vi "Collection-PED.vi"(8 "error in":errorcluster) -> (0 "error out":errorcluster)   [LabVIEW 2013]
uses:
  <vilib>/Utility/miscctls.llb/LVCursorListTypeDef.ctl
  Collection Support/Controls/PED States.ctl
  Collection Support/Controls/FirstCall.ctl
panel:
  out "Pressure Chart":dynamicdata(graph)
  out "Audio Chart":dynamicdata(graph)
  in  "Exit Button":bool
  in  "Restart Button":bool
  out "Test Type":string
  in  "Settings":bool
  in  "Trial Duration (s)":dbl=10.0 min=0.0 max=15.0 step=1.0 format="%#_13g"
  in  "Max Time":dbl=1.3 min=0.0 max=2.0 format="%#_13g"
  in  "Start Second":dbl=2.5 min=1.0 max=2.5 step=0.1 format="%#_13g"
  in  "Interruptions":i32 min=0 max=10 step=1
  in  "Delay":u32 max=1000 step=50
  in  "Min Time":dbl=0.8 min=0.0 max=1.0 step=0.1 format="%#_13g"
  out "SPL Chart":cluster{"Y":dbl[], "Y":dbl[]}[](graph)
  out "Saving Data":bool
  out "Countdown":dbl format="%#.0g"
  in  "START/STOP":bool
  in  "Stopped?":bool
  out "GO/STOP":bool
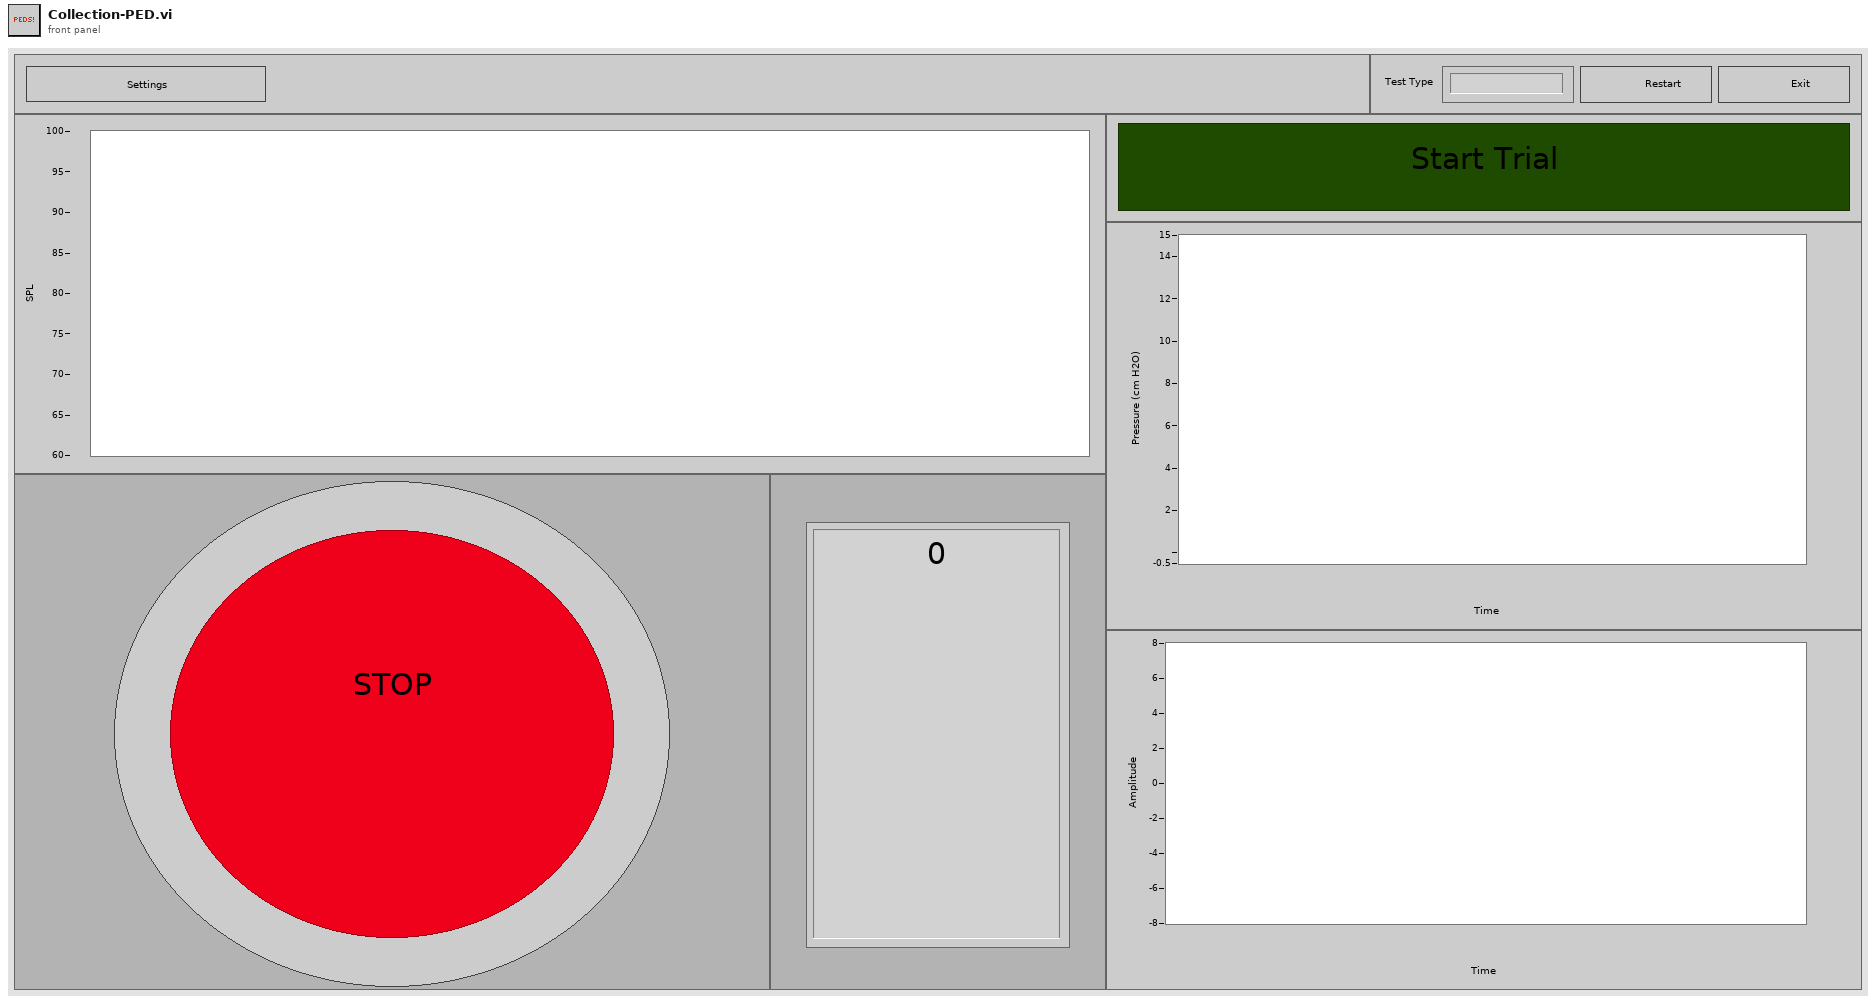
[diagram p1: front panel]
types:
  T1 = enum16{"open", "replace", "create", "open or create", "replace or create", "replace or create with confirmation"}
  T2 = typedef "LVCursorListTypeDef.ctl" = cluster{"Name":string, "Color":u32, "Style":u8, "Point Style":u8, "Name Visible":bool, "Allow Drag":bool, "Cursor Mode":u32, "Plot":i32, "Index":i32, "Position":cluster{"X":dbl, "Y":dbl}, "X Scale":u32, "Y Scale":u32, "Watch Plots":i32[], "Watch All Plots":bool, "Plot Area":i32, "Label Offset":cluster{"X":dbl, "Y":dbl}}[]
  T3 = typedef "PED States.ctl" = enum16{"Initialize", "Wait", "Record", "Save", "Reset", "Exit"}
  T4 = typedef "FirstCall.ctl" = enum16{"First", "After"}
  T5 = typedef "Mech-Labial Test Types.ctl" = u16
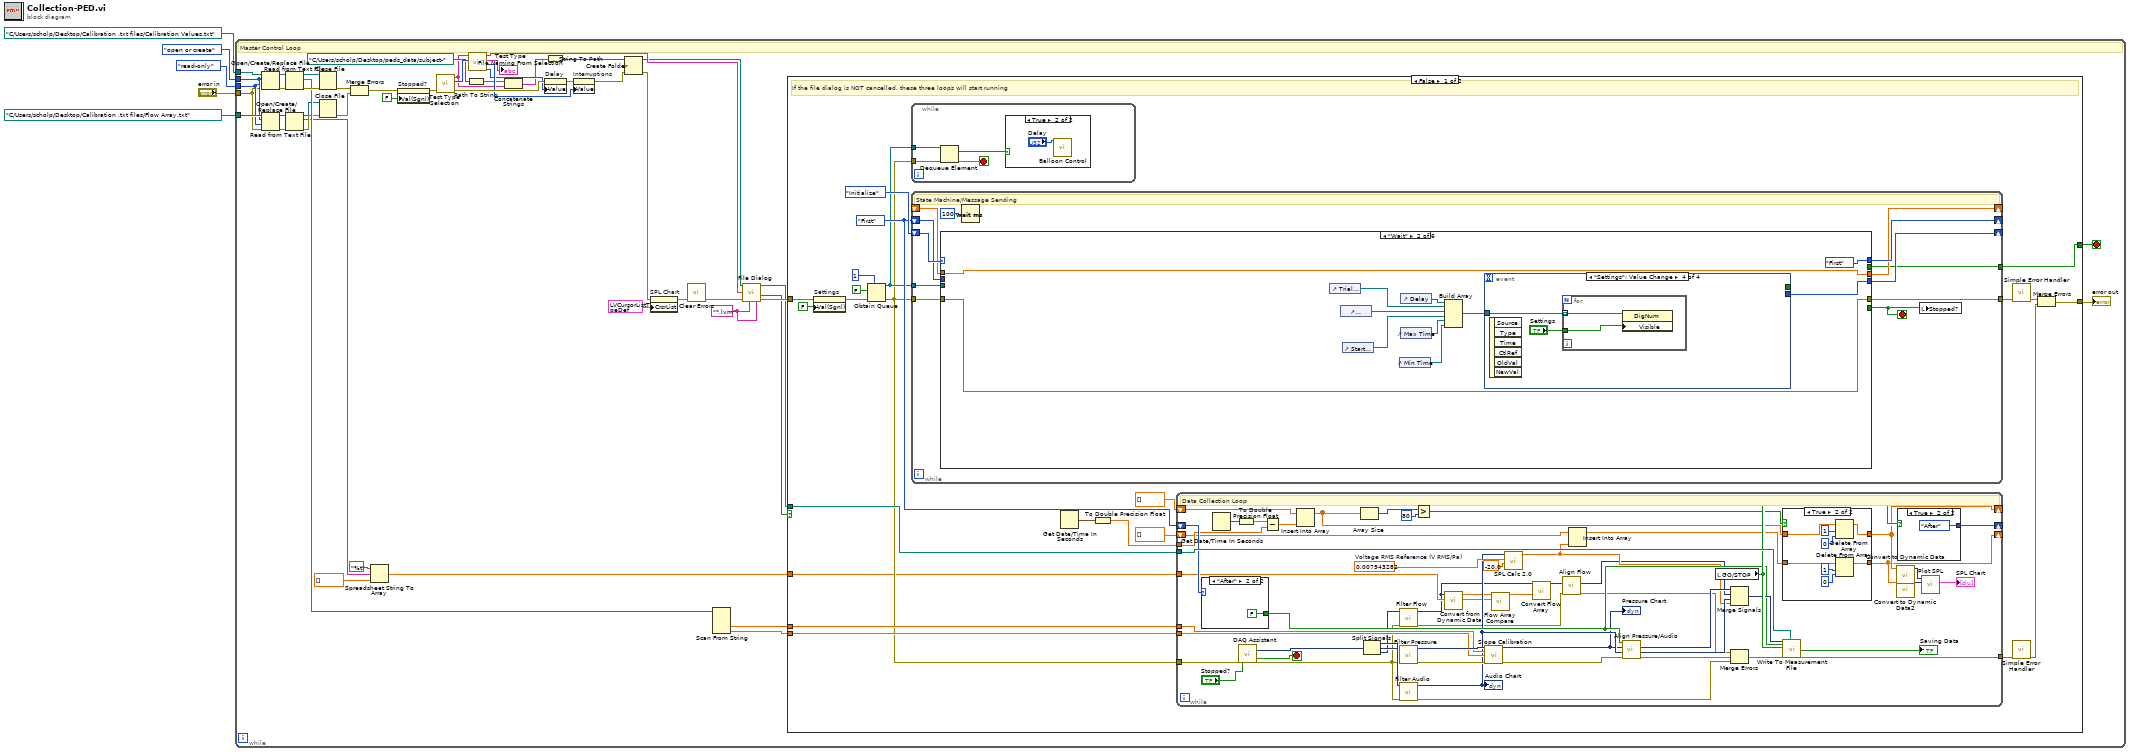
[diagram p0: block diagram]
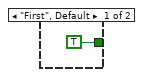
[diagram p4: hidden frame]
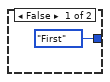
[diagram p5: hidden frame]
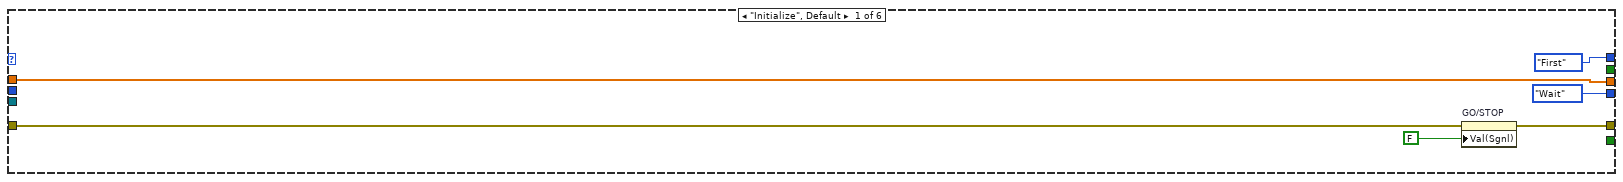
[diagram p6: hidden frame]
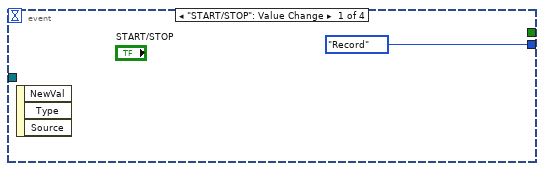
[diagram p7: hidden frame]
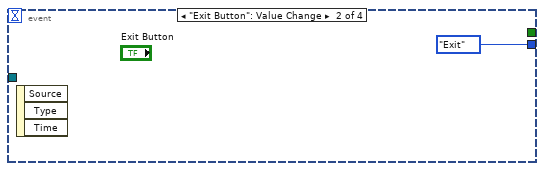
[diagram p8: hidden frame]
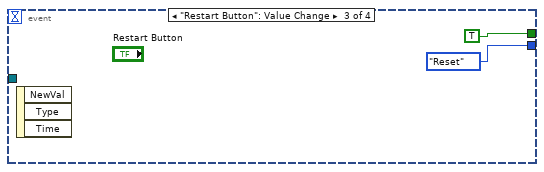
[diagram p9: hidden frame]
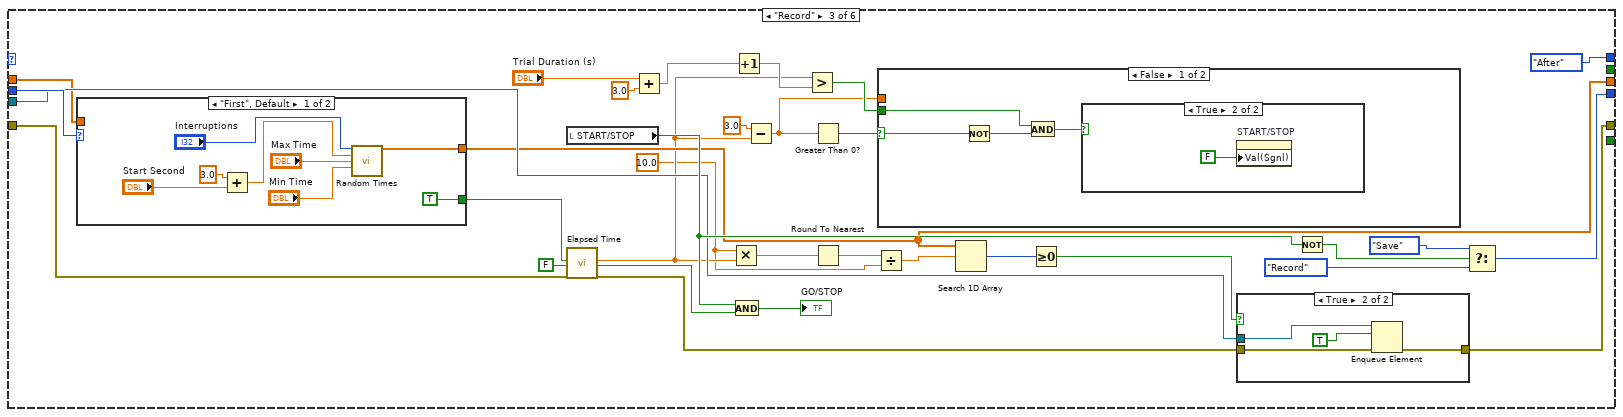
[diagram p10: hidden frame]
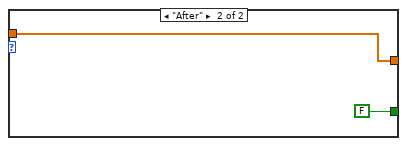
[diagram p12: hidden frame]
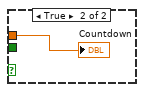
[diagram p14: hidden frame]
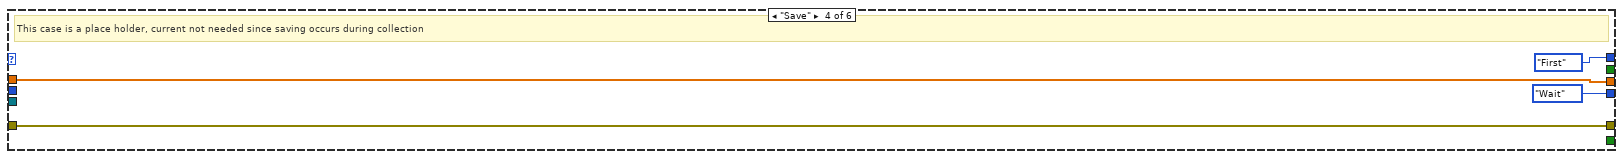
[diagram p15: hidden frame]
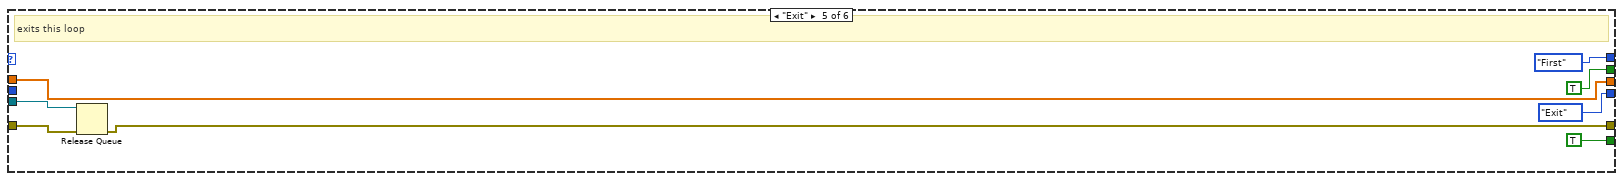
[diagram p16: hidden frame]
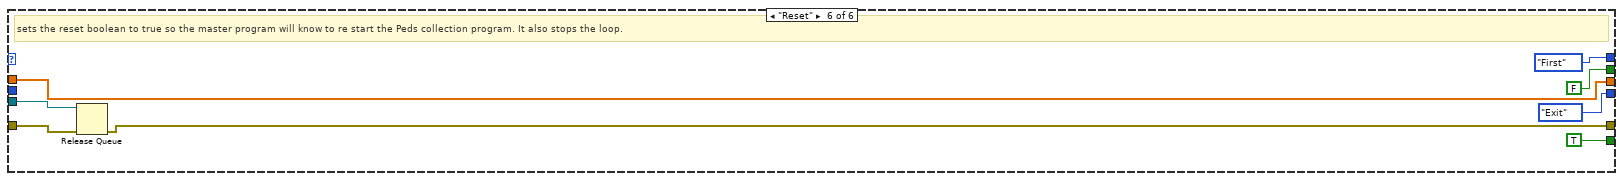
[diagram p17: hidden frame]
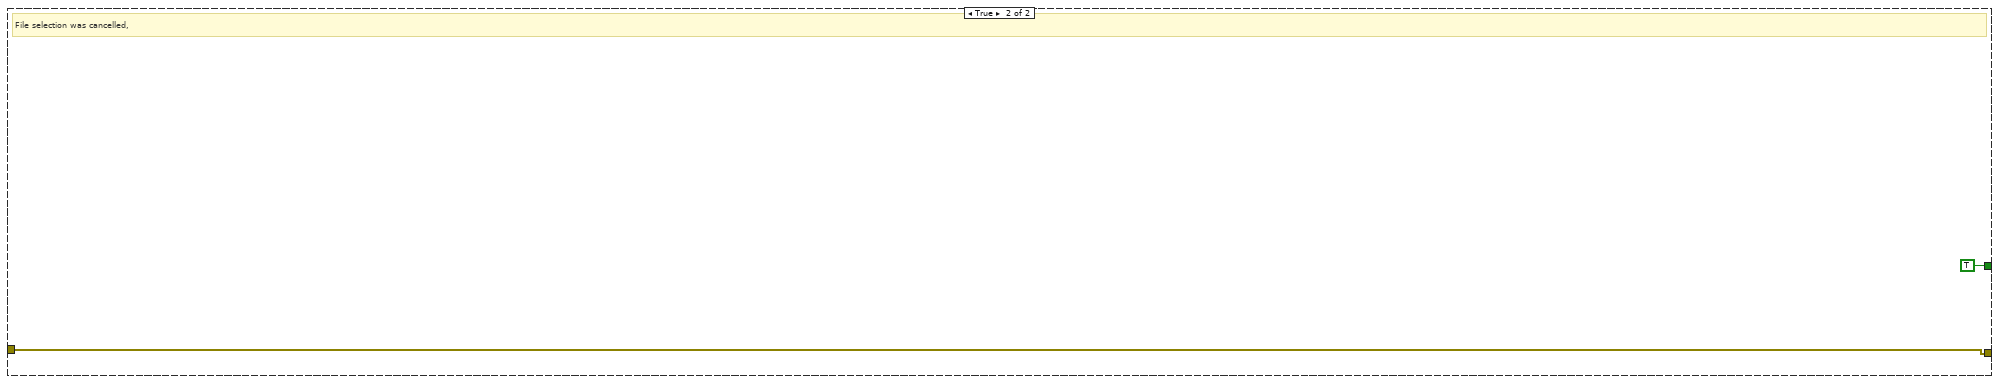
[diagram p18: hidden frame]
diagram:
  n1 = while {
    tunnel: T1."open or create" ("operation (0:open)") -> [w15]
    tunnel: enum16{"read/write", "read-only", "write-only"}."read-only" ("access (0:read/write)") -> [w14]
    tunnel: path "C:/Users/scholp/Desktop/Calibration .txt files/Calibration Values.txt" ("file path (use dialog)") -> [w47]
    tunnel: "error in" -> [w13]
    tunnel: path "C:/Users/scholp/Desktop/Calibration .txt files/Flow Array.txt" ("file path (use dialog)") -> [w16]
    stop <- w37 stop-if-true
    w52 = "*.lvm" ("pattern label")
    # "Master Control Loop"
    n2 = Open/Create/Replace File(file path (use dialog)=w47, error in=w13, operation (0:open)=w15, access (0:read/write)=w14) -> (refnum out=w48:refnum<file>, error out=w50:errorcluster)  [unwired: 2 in, 1 out]
    n3 = Open/Create/Replace File(file path (use dialog)=w16, error in=w13, operation (0:open)=w15, access (0:read/write)=w14) -> (refnum out=w18:refnum<file>, error out=w20:errorcluster)  [unwired: 2 in, 1 out]
    n4 = Read from Text File(file (use dialog)=w48, error in=w50) -> (refnum out=w46:refnum<file>, text=w45:string, error out=w49:errorcluster)  [unwired: 2 in, 1 out]
    n5 = Read from Text File(file (use dialog)=w18, error in=w20) -> (refnum out=w17:refnum<file>, text=w8:string, error out=w19:errorcluster)  [unwired: 2 in, 1 out]
    n6 = Close File(refnum=w46, error in=w49) -> (error out=w11:errorcluster)  [unwired: 1 out]
    n7 = Close File(refnum=w17, error in=w19) -> (error out=w10:errorcluster)  [unwired: 1 out]
    n8 = Merge Errors(w11, w10) -> (w12:errorcluster)
    n9 = Spreadsheet String To Array(format string="%t", spreadsheet string=w8, array type (2D Dbl)=dbl[] []) -> (array=w7:dbl[])  [unwired: 1 in]
    n10 = property on="Stopped?" class="Bool (strict)"(error in=w12, "Val(Sgnl)"=FALSE ("Value (Signaling)")) -> (error out=w40:errorcluster)  [unwired: 1 in, 1 out]
    n11 = call "Test Type Selection.vi"("Error In"=w40) -> ("Error Out"=w39:errorcluster, "Test Type Out"=w32:T5, "Subject Out"=w28:string)  [unwired: 8 in]
    n12 = Path To String(path=path "C:/Users/scholp/Desktop/peds_data/subject-" ("start path")) -> (string=w29:string)
    n13 = call "File Naming From Selection.vi"("Test Type In"=w32, "Subject In"=w28) -> ("Delay"=w33:u32, "Interruptions"=w34:u32, "Test Type"=→"Test Type":string, "File Name"=w36:string)  [unwired: 6 in]
    n14 = Concatenate Strings(w29, w28) -> (w27:string)
    n15 = property on="Delay" class="DigNum (strict)"(error in=w39, "Value"=w33) -> (error out=w38:errorcluster)  [unwired: 1 in, 1 out]
    n16 = String To Path(string=w27) -> (path=w26:path)
    n17 = property on="Interruptions" class="DigNum (strict)"(error in=w38, "Value"=w34) -> (error out=w24:errorcluster)  [unwired: 1 in, 1 out]
    n18 = Create Folder(path (use dialog)=w26, error in=w24) -> (created path=w31:path, error out=w22:errorcluster)  [unwired: 1 in, 1 out]
    n19 = property on="SPL Chart" class="XYGraph (strict)"(error in=w22, "CrsrList"=T2 [{"Name"="Upper", "Color"=16860, "Style"=6, "Point Style"=6, "Name Visible"=TRUE, "Allow Drag"=TRUE, "Cursor Mode"=0, "Plot"=0, "Index"=0, "Position"={"X"=4.012670393065205, "Y"=89.47406993320811}, "X Scale"=0, "Y Scale"=0, "Watch Plots"=[], "Watch All Plots"=FALSE, "Plot Area"=0, "Label Offset"={"X"=-0.0013496383482243246, "Y"=198885117671824.3}}, {"Name"="Lower", "Color"=6618880, "Style"=6, "Point Style"=13, "Name Visible"=TRUE, "Allow Drag"=TRUE, "Cursor Mode"=0, "Plot"=0, "Index"=0, "Position"={"X"=1.9573651669874723, "Y"=85.30922361500785}, "X Scale"=0, "Y Scale"=0, "Watch Plots"=[], "Watch All Plots"=FALSE, "Plot Area"=0, "Label Offset"={"X"=0.0011253990502635425, "Y"=1813042855982289.8}}] ("Cursor List")) -> (error out=w21:errorcluster)  [unwired: 1 in, 1 out]
    n20 = call <vilib>:"Clear Errors.vi"("error in (no error)"=w21) -> ("error out"=w25:errorcluster)  [unwired: 6 in]
    n21 = Scan From String(input string=w45) -> (output 1=w44:dbl, output 2=w43:dbl)  [unwired: 5 in, 3 out]
    n22 = call "File Dialog"("start path"=w31, "default name"=w36, "error in"=w25, "pattern (all files)"=w52, "pattern label"=w52) -> ("selected path"=w53:path, "cancelled"=w42:bool, "error out"=w54:errorcluster)  [unwired: 7 in, 1 out]
    n23 = case shown="False" w42 {
      tunnel: w54 -> [w61 w263]
      tunnel: w53 -> [w73 _]
      tunnel: w44 -> [w70 _]
      tunnel: w43 -> [w69 _]
      tunnel: [w66 w263] -> w41
      tunnel: [w65 TRUE] -> w37
      tunnel: w7 -> [w55 _]
      frame False {
        w74 = FirstCall."First"
        # "If the file dialog is NOT cancelled, these three loops will start running"
        n24 = property on="Settings" class="Bool (strict)"(error in=w61, "Val(Sgnl)"=FALSE ("Value (Signaling)")) -> (error out=w60:errorcluster)  [unwired: 1 in, 1 out]
        n25 = Obtain Queue(max queue size (-1, unlimited)=1, element data type=FALSE, error in (no error)=w60) -> (queue out=w64:refnum<queue>, error out=w63:errorcluster)  [unwired: 2 in, 1 out]
        n26 = while {
          tunnel: w64 -> [w81]
          tunnel: w63 -> [w80]
          stop <- w79 stop-if-true
          n27 = Dequeue Element(queue=w81, error in (no error)=w80) -> (element=w78:bool, error out=w79:errorcluster)  [unwired: 1 in, 2 out]
          n28 = case shown="True" w78 {
            frame False {
            }
            frame True {
              n29 = call "Balloon Control.vi"("Delay (ms)"="Delay") -> ()  [unwired: 11 in]
            }
          }
        }
        n30 = while {
          shift-right: [w163] -> _
          shift-left: PED_States."Initialize" -> [w162]
          tunnel: w64 -> [w159]
          tunnel: w63 -> [w161]
          shift-right: [w158] -> _
          shift-left: w74 -> [w160]
          tunnel: [w156] -> w71
          shift-right: [w153] -> _
          shift-left: _ -> [w154]
          tunnel: [w152] -> w65
          stop <- w157 stop-if-true
          # "State Machine/Message Sending"
          n31 = case shown="\"Wait\"" w162 {
            tunnel: [_ _ _ _ TRUE TRUE] -> w157
            tunnel: [PED_States."Wait" ("f") w180 w205 PED_States."Wait" ("element") PED_States."Exit" ("element") PED_States."Exit" ("element")] -> w163
            tunnel: w161 -> [w164 w177 w211 w243 w251 w256]
            tunnel: w160 -> [_ _ w207 _ _ _]
            tunnel: w159 -> [_ _ w202 _ w250 w255]
            tunnel: [FirstCall."First" FirstCall."First" FirstCall."After" FirstCall."First" FirstCall."First" FirstCall."First"] -> w158
            tunnel: [w167 w178 w199 w242 w247 w261] -> w153
            tunnel: [w165 w177 w201 w243 w248 w257] -> w156
            tunnel: w154 -> [w167 w178 w198 w242 w247 w261]
            tunnel: [_ _ _ _ TRUE FALSE] -> w152
            frame "Initialize", Default {
              n32 = property on="GO/STOP" class="Bool (strict)"(error in=w164, "Val(Sgnl)"=FALSE ("Value (Signaling)")) -> (error out=w165:errorcluster)  [unwired: 1 in, 1 out]
            }
            frame "Wait" {
              n33 = control-ref of="Trial Duration (s)"() -> (w172:refnum<vi>)
              n34 = control-ref of="Interruptions"() -> (w173:refnum<vi>)
              n35 = control-ref of="Start Second"() -> (w174:refnum<vi>)
              n36 = control-ref of="Min Time"() -> (w176:refnum<vi>)
              n37 = control-ref of="Delay"() -> (w171:refnum<vi>)
              n38 = control-ref of="Max Time"() -> (w175:refnum<vi>)
              n39 = Build Array(w171, w172, w173, w174, w175, w176) -> (w170:refnum<vi>[])
              n40 = event shown="[3] \"Settings\": Value Change" {
                selector: _ -> [_ _ _ _]
                dyn-events: _ -> [_ _ _ _]
                timeout: _ -> [_ _ _ _]
                tunnel: [PED_States."Record" ("element") PED_States."Exit" ("element") PED_States."Reset" ("element") _] -> w180
                tunnel: [_ _ TRUE _] -> _
                tunnel: w170 -> [_ _ _ w186]
                event "START/STOP": Value Change {
                  n41 = event-data() -> ()  [unwired: 1 in, 3 out]
                }
                event "Exit Button": Value Change {
                  n42 = event-data() -> ()  [unwired: 1 in, 3 out]
                }
                event "Restart Button": Value Change {
                  n43 = event-data() -> ()  [unwired: 1 in, 3 out]
                }
                event "Settings": Value Change {
                  n44 = event-data() -> ()  [unwired: 1 in, 6 out]
                  n45 = for {
                    tunnel: w186 -> [w188] mode=indexing
                    tunnel: "Settings" -> [w187]
                    n46 = property class="DigNum"(reference=w188, "Visible"=w187) -> ()  [unwired: 1 in, 2 out]
                  }
                }
              }
            }
            frame "Record" {
              w190 = 10.0 ("x")
              n47 = case shown="\"First\", Default" w207 {
                tunnel: [TRUE FALSE] -> w208
                tunnel: [w230 w234] -> w199
                tunnel: w198 -> [_ w234]
                frame "First", Default {
                  n48 = Add(x=3.0, y="Start Second") -> (x+y=w228:dbl)
                  n49 = call "Random Times.vi"("Number of Interruptions"="Interruptions", "Start Second"=w228, "Longest Gap"="Max Time", "Shortest Gap"="Min Time") -> ("Interruption TImes"=w230:dbl[])  [unwired: 10 in, 1 out]
                }
                frame "After" {
                }
              }
              n50 = local read "START/STOP"() -> (w212:bool)
              n51 = call "Elapsed Time"("Reset"=w208, "Auto Reset"=FALSE, "error in (no error)"=w211) -> ("Elapsed Time (s)"=w192:dbl, "Time has Elapsed"=w214:bool, "error out"=w203:errorcluster)  [unwired: 9 in, 5 out]
              n52 = Add(x="Trial Duration (s)", y=3.0) -> (x+y=w195:dbl)
              n53 = Multiply(x=w190, y=w192) -> (x*y=w193:dbl)
              n54 = And(x=w212, y=w214) -> (x .and. y?=→"GO/STOP":bool)
              n55 = Increment(x=w195) -> (x+1=w197:dbl)
              n56 = Subtract(x=3.0, y=w192) -> (x-y=w215:dbl)
              n57 = Greater?(x=w192, y=w197) -> (0:w217:bool)
              n58 = Greater Than 0?(x=w215) -> (x > 0?=w218:bool)
              n59 = Round To Nearest(number=w193) -> (nearest integer value=w191:dbl)
              n60 = Divide(x=w191, y=w190) -> (x/y=w189:dbl)
              n61 = case shown="False" w218 {
                selector: w218 -> [w237 _]
                tunnel: w215 -> [_ w241]
                tunnel: w217 -> [w239 _]
                frame False {
                  n62 = Not(x=w237) -> (.not. x?=w236:bool)
                  n63 = And(x=w239, y=w236) -> (x .and. y?=w238:bool)
                  n64 = case shown="True" w238 {
                    frame False {
                    }
                    frame True {
                      n65 = property on="START/STOP" class="Bool (strict)"("Val(Sgnl)"=FALSE ("Value (Signaling)")) -> ()  [unwired: 2 in, 2 out]
                    }
                  }
                }
                frame True {
                  "Countdown" <- w241
                }
              }
              n66 = Search 1D Array(1D array=w199, element=w189) -> (index of element=w204:i32)  [unwired: 1 in]
              n67 = Greater Or Equal To 0?(x=w204) -> (x >= 0?=w200:bool)
              n68 = case shown="True" w200 {
                tunnel: [w221 w225] -> w201
                tunnel: w203 -> [w221 w224]
                tunnel: w202 -> [_ w223]
                frame False {
                }
                frame True {
                  n69 = Enqueue Element(queue=w223, element=TRUE, error in (no error)=w224) -> (error out=w225:errorcluster)  [unwired: 1 in, 2 out]
                }
              }
              n70 = Not(x=w212) -> (.not. x?=w210:bool)
              n71 = Select(t=PED_States."Save" ("f"), s=w210, f=PED_States."Record") -> (s? t:f=w205:T3)
            }
            frame "Save" {
              # "This case is a place holder, current not needed since saving occurs during collection"
            }
            frame "Exit" {
              # "exits this loop"
              n72 = Release Queue(queue=w250, error in (no error)=w251) -> (error out=w248:errorcluster)  [unwired: 1 in, 2 out]
            }
            frame "Reset" {
              # "sets the reset boolean to true so the master program will know to re start the Peds collection program. It also stops the loop."
              n73 = Release Queue(queue=w255, error in (no error)=w256) -> (error out=w257:errorcluster)  [unwired: 1 in, 2 out]
            }
          }
          n74 = Wait (ms)(milliseconds to wait=u32 100) -> ()  [unwired: 1 out]
          n75 = local write "Stopped?"(w157) -> ()
        }
        n76 = Get Date/Time In Seconds() -> (seconds since 1Jan1904=w59:timestamp)
        n77 = To Double Precision Float(number=w59) -> (double precision float=w58:dbl)
        n78 = while {
          tunnel: w63 -> [w134]
          shift-right: [w132] -> _
          shift-left: w74 -> [w127]
          tunnel: w73 -> [w129]
          tunnel: [w128] -> w72
          tunnel: w70 -> [w131]
          tunnel: w69 -> [w130]
          tunnel: w58 -> [w106]
          shift-right: [w102] -> _
          shift-left: dbl[] [] -> [w105]
          shift-right: [w96] -> _
          shift-left: dbl[] [] -> [w103]
          tunnel: w55 -> [w88]
          stop <- w135 stop-if-true
          w113 = 0.007943282  # Voltage RMS Reference (V RMS/Pa)
          # "Data Collection Loop"
          n79 = case shown="\"After\"" w127 {
            tunnel: [TRUE FALSE] -> w114
            frame "First", Default {
            }
            frame "After" {
            }
          }
          n80 = Get Date/Time In Seconds() -> (seconds since 1Jan1904=w110:timestamp)
          n81 = To Double Precision Float(number=w110) -> (double precision float=w107:dbl)
          n82 = call "DAQ Assistant"("error in"=w134, "stop (F)"="Stopped?") -> ("data"=w124:dynamicdata, "stopped"=w135:bool, "error out"=w92:errorcluster)  [unwired: 14 in, 1 out]
          n83 = Subtract(x=w107, y=w106) -> (x-y=w104:dbl)
          n84 = Insert Into Array(array=w105, new element=w104) -> (w101:dbl[])  [unwired: 1 in]
          n85 = Array Size(array=w101) -> (size(s)=w98:i32)
          n86 = Split Signals(w124) -> (w123:dynamicdata, w122:dynamicdata, w93:dynamicdata)  [unwired: 3 in]
          n87 = call "Filter Flow"("error in (no error)"=w92, "Signal"=w93) -> ("error out"=w84:errorcluster, "Filtered Signal"=w87:dynamicdata)  [unwired: 8 in]
          n88 = call "Filter Pressure"("error in (no error)"=w92, "Signal"=w122) -> ("error out"=w136:errorcluster, "Filtered Signal"=w137:dynamicdata)  [unwired: 8 in]
          n89 = call "Filter Audio"("error in (no error)"=w92, "Signal"=w123) -> ("error out"=w118:errorcluster, "Filtered Signal"=w95:dynamicdata)  [unwired: 8 in]
          "Audio Chart" <- w95
          n90 = Greater?(x=w98, y=80) -> (0:w99:bool)
          n91 = call "Convert from Dynamic Data"("Dynamic Data Type"=w87) -> ("Array"=w89:dbl[])  [unwired: 3 in]
          n92 = call "Slope Calibration.vi"("Voltage"=w137, "Slope"=w131, "Intercept"=w130, "error in (no error)"=w136) -> ("Result"=w94:dynamicdata, "error out"=w120:errorcluster)  [unwired: 10 in]
          "Pressure Chart" <- w94
          n93 = call "Flow Array Compare.vi"("Flow Array in"=w88, "Array in"=w89) -> ("Array out"=w90:dbl[])  [unwired: 9 in]
          n94 = call "SPL Calc 2.0.vi"("Gain"=-20.0, "Voltage RMS Reference (V RMS/Pa)"=w113, "Dynamic Data"=w95) -> ("SPL"=w91:dbl)  [unwired: 8 in]
          n95 = call "Convert Flow Array.vi"("Voltage"=w87, "Array - Numeric"=w90) -> ("Result"=w86:dynamicdata)  [unwired: 12 in, 1 out]
          n96 = call "Align Flow"("error in (no error)"=w84, "Signals"=w86) -> ("error out"=w83:errorcluster, "Resampled Signals"=w85:dynamicdata)  [unwired: 7 in, 1 out]
          n97 = Insert Into Array(array=w103, new element=w91) -> (w97:dbl[])  [unwired: 1 in]
          n98 = call "Align Pressure/Audio"("error in (no error)"=w120, "Signals 2"=w95, "Signals"=w94, "Reset"=w114) -> ("error out"=w119:errorcluster, "Resampled Signals 2"=w117:dynamicdata, "Resampled Signals"=w121:dynamicdata)  [unwired: 5 in]
          n99 = local read "GO/STOP"() -> (w125:bool)
          n100 = Merge Signals(w121, w85, w117, w91) -> (w116:dynamicdata)
          n101 = Merge Errors(w83, w119, w118) -> (w115:errorcluster)
          n102 = case shown="True" w99 {
            tunnel: w101 -> [w139 w147]
            tunnel: [w139 w146] -> w102
            tunnel: w97 -> [w138 w141]
            tunnel: [w138 w140] -> w96
            frame False {
            }
            frame True {
              n103 = Delete From Array(array=w147, length=1, index=0) -> (array with subset deleted=w146:dbl[])  [unwired: 1 out]
              n104 = Delete From Array(array=w141, length=1, index=0) -> (array with subset deleted=w140:dbl[])  [unwired: 1 out]
            }
          }
          n105 = call "Write To Measurement File"("Signals"=w116, "Reset"=w114, "Enable"=w125, "error in (no error)"=w115, "Filename"=w129) -> ("Saving Data"=→"Saving Data":bool, "error out"=w128:errorcluster)  [unwired: 12 in, 1 out]
          n106 = call "Convert to Dynamic Data"("Array"=w102) -> ("Dynamic Data Type"=w108:dynamicdata)  [unwired: 3 in]
          n107 = call "Convert to Dynamic Data2"("Array"=w96) -> ("Dynamic Data Type"=w109:dynamicdata)  [unwired: 3 in]
          n108 = case shown="True" w125 {
            tunnel: [FirstCall."First" FirstCall."After"] -> w132
            frame False {
            }
            frame True {
            }
          }
          n109 = call "Plot SPL"("Y Input"=w109, "X Input"=w108) -> ("XY Graph"=→"SPL Chart":cluster{"Y":dbl[], "Y":dbl[]}[])  [unwired: 8 in, 1 out]
        }
        n110 = call <vilib>:"Simple Error Handler.vi"("error in (no error)"=w71) -> ("error out"=w68:errorcluster)  [unwired: 4 in, 4 out]
        n111 = call <vilib>:"Simple Error Handler.vi"("error in (no error)"=w72) -> ("error out"=w67:errorcluster)  [unwired: 4 in, 4 out]
        n112 = Merge Errors(w68, w67) -> (w66:errorcluster)
      }
      frame True {
        # "File selection was cancelled,"
      }
    }
    "error out" <- w41
  }
